vi "DepthSense NewFrame Callback With Globals.vi"(4 "User Parameter":variant, 6 "Control Ref":refnum<k24>, 7 "Event Common Data":T1) -> ()   [LabVIEW 2011]
uses:
  C:/Users/Behavior Room/Desktop/Kinect Mouse/DepthSense/FunctionPointerProxy/FunctionPointerProxy/bin/Release/FunctionPointerProxy.dll
  FunctionPointerProxy/FunctionPointerProxy/bin/Release/FunctionPointerProxy.dll
  DepthSense Global Status.vi
  <userlib>/libOptrima-2-3/libOptrima-2-3.lvlib
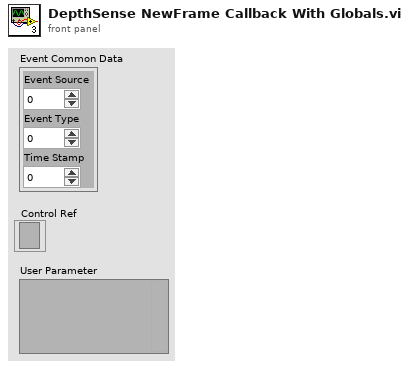
[diagram p1: front panel]
types:
  T1 = cluster{"Event Source":i32, "Event Type":u32, "Time Stamp":u32}
  T2 = typedef "Image Type" = u32
  T3 = cluster{"Camera Version":string, "Image Height":i32, "Image Width":i32, "Minimum Framerate":i32, "Maximum Framerate":i32, "Framerate":i32, "Close Mode":bool, "Denoising":bool, "Leakage Algorithm":bool, "Anti-Aliasing":bool, "Camera Status":i32, "API Version":string, "Light Intensity":i32, "Confidence Threshold":u16}
  T4 = typedef "IMAQ Image.ctl" = refnum<image>
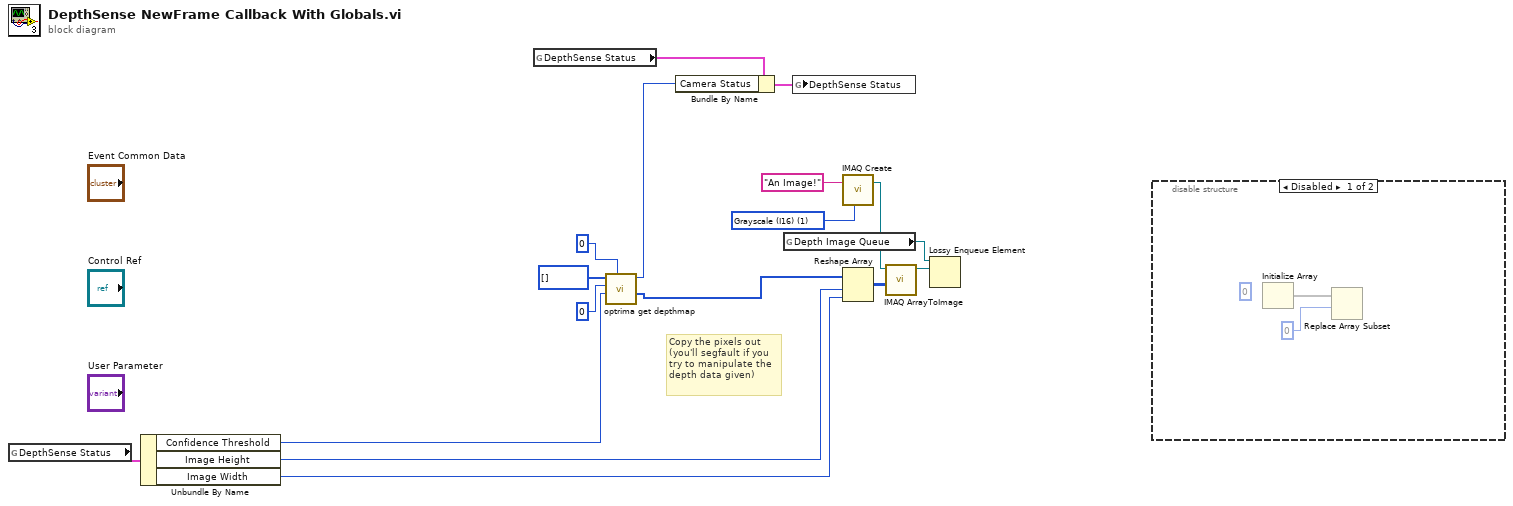
[diagram p0: block diagram]
diagram:
  w6 = T2 1 items=["Grayscale (U8)", "Grayscale (I16)", "Grayscale (SGL)", "Complex (CSG)", "RGB (U32)", "HSL (U32)", "RGB (U64)", "Grayscale (U16)"] ("Image Type")
  # "Copy the pixels out\n(you'll segfault if you\ntry to manipulate the\ndepth data given)"
  n1 = global read "DepthSense Global Status.vi" "DepthSense Status"() -> (w17:T3)
  n2 = Unbundle By Name(w17) -> ("Confidence Threshold"=w14:u16, "Image Height"=w16:i32, "Image Width"=w15:i32)
  n3 = global read "DepthSense Global Status.vi" "DepthSense Status"() -> (w13:T3)
  n4 = call <userlib>:"optrima get depthmap.vi"("to_camera_plane"=0, "confidenceTH"=w14, "length"=u32 0, "p_depthmap in"=u16[] []) -> ("p_depthmap out"=w1:u16[], "function return"=w8:u32)  [unwired: 4 in, 2 out]
  n5 = Bundle By Name(cluster=w13, "Camera Status"=w8) -> (w12:T3)
  n6 = global read "DepthSense Global Status.vi" "Depth Image Queue"() -> (w3:refnum<queue>)
  n7 = global write "DepthSense Global Status.vi" "DepthSense Status"(w12) -> ()
  n8 = call "IMAQ Create"("Image Name"="An Image!", "Image Type"=w6) -> ("New Image"=w7:T4)  [unwired: 3 in, 1 out]
  n9 = Reshape Array(w1, w16, w15) -> (w4:u16[][])
  n10 = call "IMAQ ArrayToImage"("Image Pixels (I16)"=w4, "Image"=w7) -> ("Image Out"=w2:T4)  [unwired: 8 in, 1 out]
  n11 = Lossy Enqueue Element(queue=w3, element=w2) -> ()  [unwired: 1 in, 4 out]
  n12 = disable-structure shown="Disabled" {
    frame Disabled {
      (unwired) u16 0 ("element")
      n13 = Initialize Array() -> (w20:void[])  [unwired: 2 in]
      n14 = Replace Array Subset(array=w20, index=0) -> (w18:void[])  [unwired: 1 in]
    }
    frame Enabled {
    }
  }
